vi "DSF.Engine.Framework.Rx.vi"(8 "error in (no error)":errorcluster, 11 "Framework in":refnum<class "DSF.Engine.Framework.lvclass">) -> (0 "error out":errorcluster, 3 "Framework out":refnum<class "DSF.Engine.Framework.lvclass">)   [LabVIEW 2017, in "DSF.Engine.lvlib" / "DSF.Engine.Framework.lvclass"]
uses:
  DSF.Engine.Framework.lvclass
  DSF.Engine.Framework.lvclass/DSF.Engine.Framework.ctl
  Plugin/DSF.Engine.Plugin.lvclass
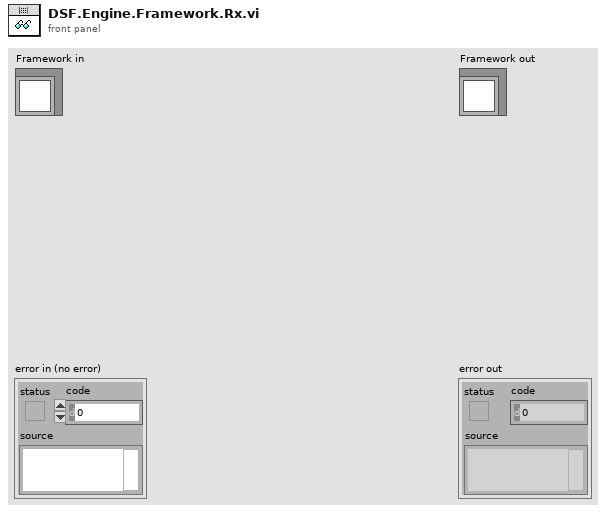
[diagram p1: front panel]
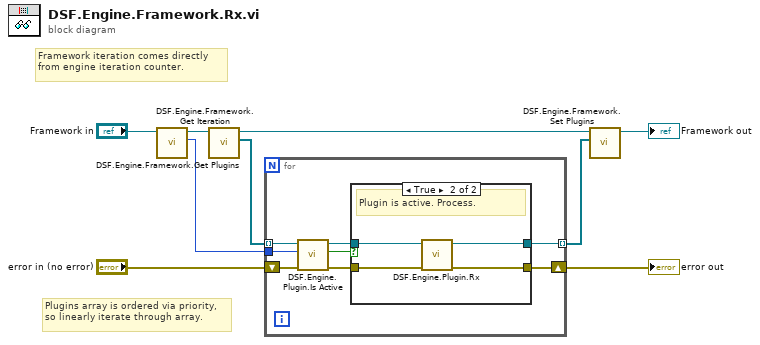
[diagram p0: block diagram]
diagram:
  # "Framework iteration comes directly from engine iteration counter."
  # "Plugins array is ordered via priority, so linearly iterate through array."
  n1 = call "DSF.Engine.Framework.Get Iteration.vi"("Framework in"="Framework in") -> ("iteration"=w6:u64, "Framework out"=w7:refnum<class "DSF.Engine.Framework.lvclass">)  [unwired: 9 in]
  n2 = call "DSF.Engine.Framework.Get Plugins.vi"("Framework in"=w7) -> ("Plugins"=w9:refnum<class "DSF.Engine.Plugin.lvclass">[], "Framework out"=w1:refnum<class "DSF.Engine.Framework.lvclass">)  [unwired: 9 in]
  n3 = for {
    tunnel: w9 -> [w16] mode=indexing
    tunnel: w6 -> [w10]
    tunnel: [w13] -> w4 mode=indexing
    shift-right: [w12] -> w2
    shift-left: "error in (no error)" -> [w11]
    n4 = call "DSF.Engine.Plugin.Is Active.vi"("cycle count"=w10, "Plugin in"=w16) -> ("active this cycle?"=w15:bool, "Plugin out"=w14:refnum<class "DSF.Engine.Plugin.lvclass">)  [unwired: 8 in]
    n5 = case shown="True" w15 {
      tunnel: w14 -> [w18 w22]
      tunnel: [w18 w20] -> w13
      tunnel: [w17 w19] -> w12
      tunnel: w11 -> [w17 w21]
      frame False {
        # "Plugin is not active. Skip."
      }
      frame True {
        # "Plugin is active. Process."
        n6 = call "DSF.Engine.Plugin.Rx.vi"("error in (no error)"=w21, "Plugin in"=w22) -> ("error out"=w19:errorcluster, "Plugin out"=w20:refnum<class "DSF.Engine.Plugin.lvclass">)  [unwired: 8 in]
      }
    }
  }
  "error out" <- w2
  n7 = call "DSF.Engine.Framework.Set Plugins.vi"("Plugins"=w4, "Framework in"=w1) -> ("Framework out"=→"Framework out":refnum<class "DSF.Engine.Framework.lvclass">)  [unwired: 9 in]
